vi "Motion_Write Axis Home Data.vi"(8 "error in":errorcluster, 9 "Register":T2=44 items=["GANTRY_MOTION"=20, "X_HOME"=40, "Y_HOME"=64, "Z_HOME"=88, "LOADER_HOME"=112, "LOADER_DIRECTION"=144], 10 "Home Data":T1 {"Position" format="%_7g"; "AccDec" format="%_7g"; "OffsetVelocity" format="%_7g"; "Offset" format="%_7g"; "Creep Velocity" format="%_7g"; "Approach Velocity" format="%_7g"}, 11 "TCP Connection Refnum in":refnum<k5>) -> (0 "error out":errorcluster, 3 "TCP Connection Refnum (dup)":refnum<k5>)   [LabVIEW 2010]
uses:
  Motion_Registers Typedef.ctl
  <vilib>/NI Modbus.llb/MB Ethernet Master Query Write Multiple Registers (poly).vi
panel:
  out "Exception Code":u8 format="%.0x"
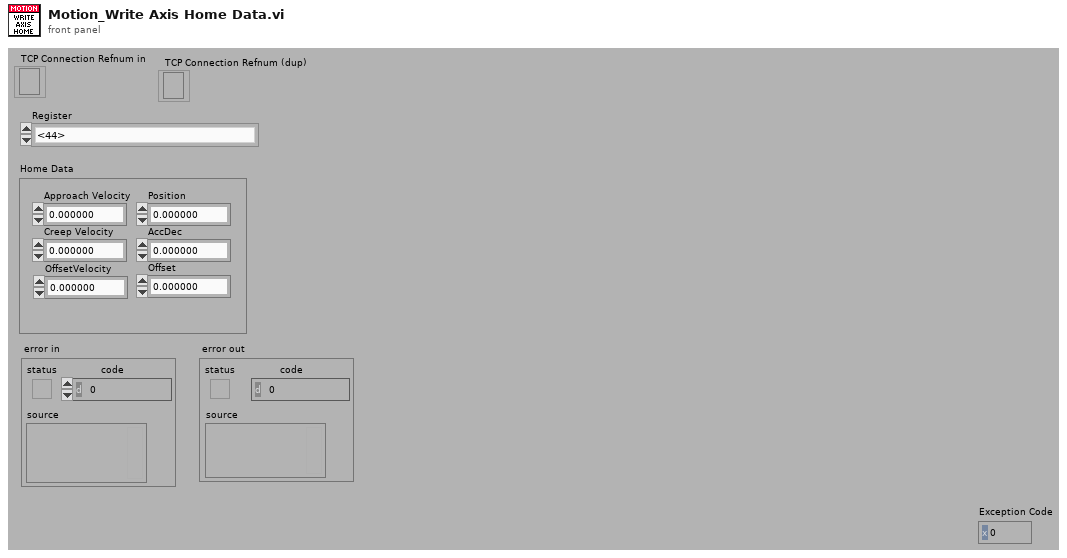
[diagram p1: front panel]
types:
  T1 = cluster{"Approach Velocity":dbl, "Creep Velocity":dbl, "Offset":dbl, "OffsetVelocity":dbl, "AccDec":dbl, "Position":dbl}
  T2 = typedef "Motion_Registers Typedef.ctl" = u16
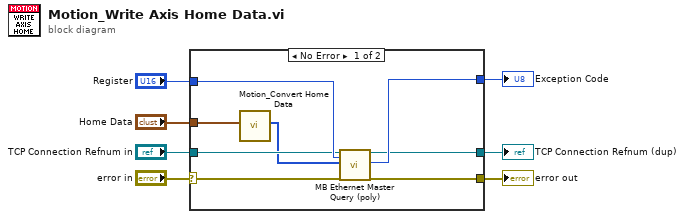
[diagram p0: block diagram]
diagram:
  n1 = case shown="No Error" "error in" {
    selector: "error in" -> [w8 w17]
    tunnel: "Register" -> [w15 _]
    tunnel: [w14 _] -> w6
    tunnel: "Home Data" -> [w13 _]
    tunnel: [w12 w17] -> w4
    tunnel: "TCP Connection Refnum in" -> [w11 w16]
    tunnel: [w10 w16] -> w2
    frame No Error {
      n2 = call "Motion_Convert Home Data.vi"("Home Data"=w13) -> ("Home Data"=w9:u16[])  [unwired: 10 in]
      n3 = call-poly <vilib>:"MB Ethernet Master Query (poly).vi"("TCP Connection Refnum in"=w11, "Starting Address"=w15, "Registers"=w9, "error in"=w8) -> ("TCP Connection Refnum (dup)"=w10:refnum<k5>, "Exception Code"=w14:u8, "error out"=w12:errorcluster)  [unwired: 13 in]
    }
    frame Error {
    }
  }
  "Exception Code" <- w6
  "error out" <- w4
  "TCP Connection Refnum (dup)" <- w2
